vi "isoObject_client.vi"() -> ()   [LabVIEW 2021]
panel:
  out "data out":string
  out "connection ID":refnum<k5>
  out "error out":errorcluster
  in  "address":string
  in  "remote port or service name":u16
  in  "timeout ms":i32
  in  "error in (no error)":errorcluster
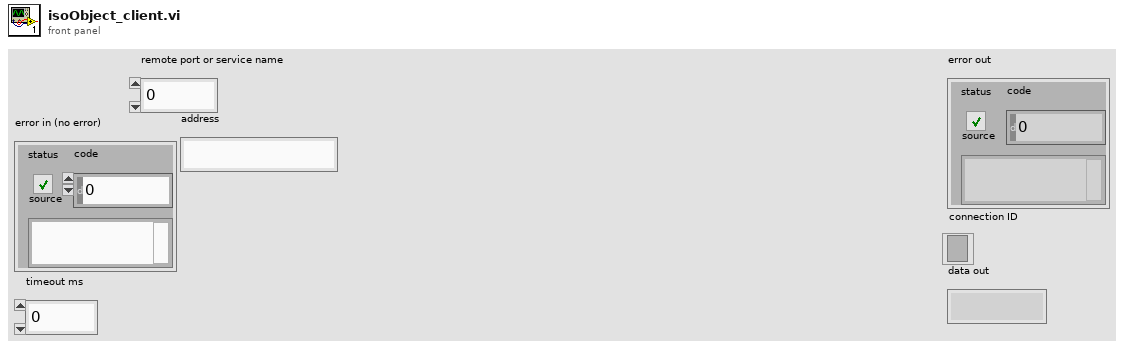
[diagram p1: front panel]
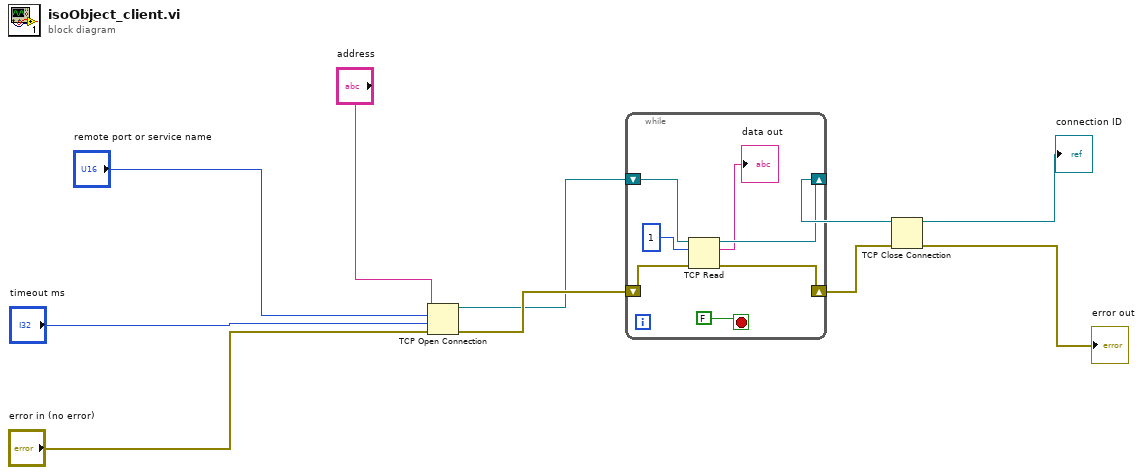
[diagram p0: block diagram]
diagram:
  n1 = TCP Open Connection(address="address", remote port or service name="remote port or service name", timeout ms (60000)="timeout ms", error in (no error)="error in (no error)") -> (connection ID=w5:refnum<k5>, error out=w6:errorcluster)  [unwired: 1 in]
  n2 = while {
    shift-right: [w14] -> w3
    shift-left: w6 -> [w15]
    shift-right: [w13] -> w4
    shift-left: w5 -> [w16]
    stop <- FALSE stop-if-true
    n3 = TCP Read(connection ID=w16, bytes to read=1, error in (no error)=w15) -> (connection ID out=w13:refnum<k5>, data out=→"data out":string, error out=w14:errorcluster)  [unwired: 2 in]
  }
  n4 = TCP Close Connection(connection ID=w4, error in (no error)=w3) -> (connection ID out=→"connection ID":refnum<k5>, error out=→"error out":errorcluster)  [unwired: 1 in]
